vi "Sensor Interface.vi"(8 "Error In":errorcluster) -> (0 "Error Out":errorcluster)   [LabVIEW 2017]
panel:
  in  "Elevator Position":u32(slide) scale=1.0..4.0
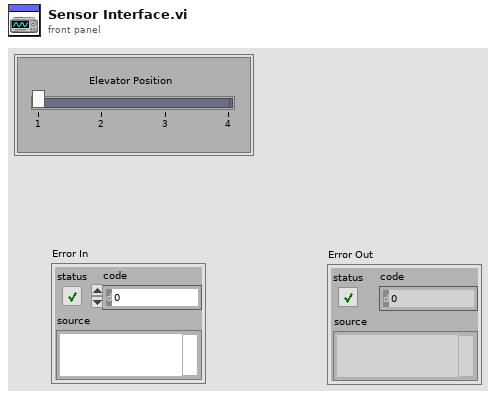
[diagram p1: front panel]
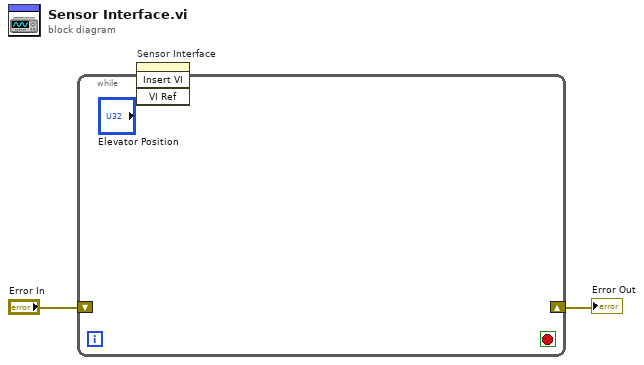
[diagram p0: block diagram]
diagram:
  n1 = while {
    shift-right: [_] -> w1
    shift-left: "Error In" -> [_]
    stop <- _ stop-if-true
  }
  "Error Out" <- w1
  n2 = invoke on="Sensor Interface" class="SubPnl" method="Insert VI"() -> ()  [unwired: 4 in, 4 out]
